vi "ReactorInitialization.vi"(1 "Reactor Selector":T2(ring)) -> (0 "System Constants":T1)   [LabVIEW 2022 SP3]
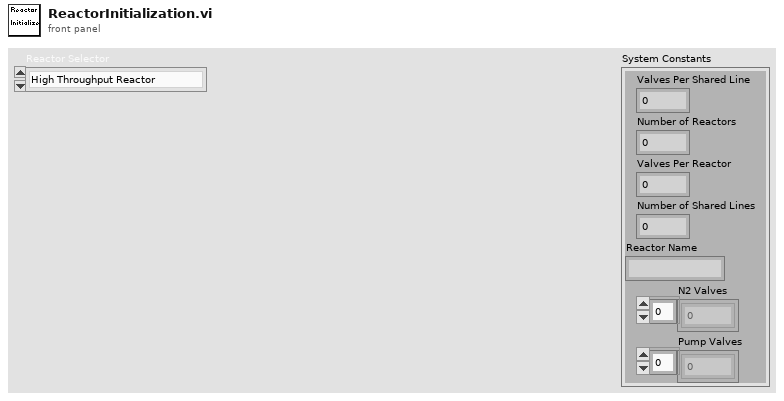
[diagram p1: front panel]
types:
  T1 = cluster{"Valves Per Shared Line":i32, "Number of Reactors":i32, "Valves Per Reactor":i32, "Number of Shared Lines":i32, "Reactor Name":string, "N2 Valves":i32[], "Pump Valves":i32[]}
  T2 = enum16{"High Throughput Reactor", "In Situ Reactor", "MLD Reactor"}
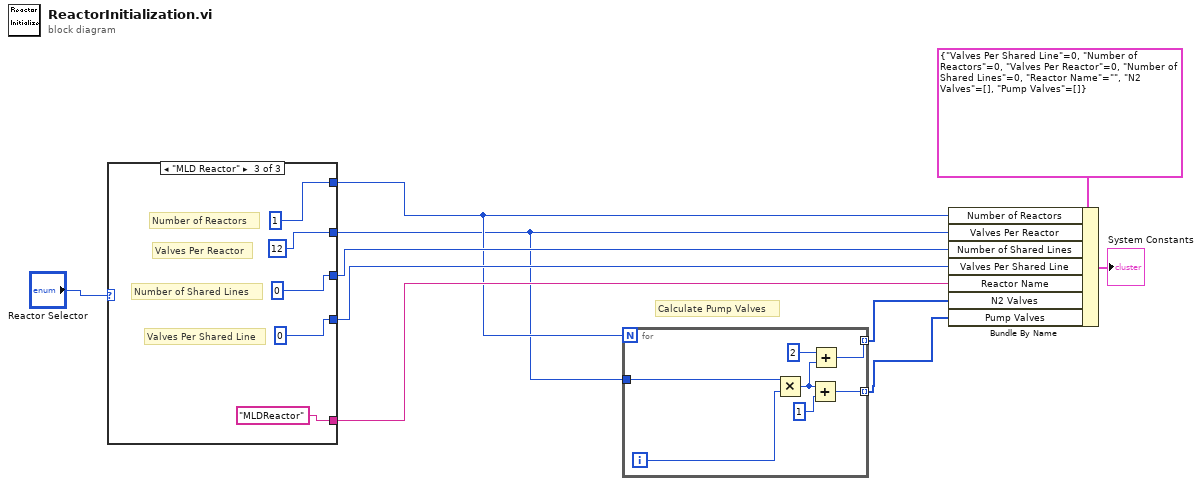
[diagram p0: block diagram]
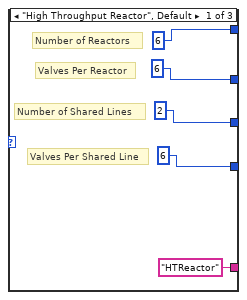
[diagram p2: hidden frame]
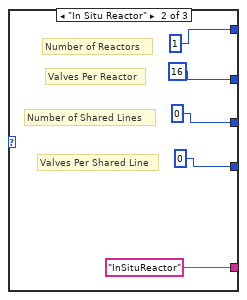
[diagram p3: hidden frame]
diagram:
  # "Calculate Pump Valves"
  n1 = case shown="\"MLD Reactor\"" "Reactor Selector" {
    tunnel: [6 1 1] -> w2
    tunnel: [6 16 12] -> w1
    tunnel: [2 0 0] -> w5
    tunnel: [6 0 0] -> w4
    tunnel: ["HTReactor" ("Reactor Name") "InSituReactor" ("Reactor Name") "MLDReactor" ("Reactor Name")] -> w3
    frame "High Throughput Reactor", Default {
      # "Valves Per Shared Line"
      # "Number of Shared Lines"
      # "Valves Per Reactor"
      # "Number of Reactors"
    }
    frame "In Situ Reactor" {
      # "Valves Per Shared Line"
      # "Number of Shared Lines"
      # "Valves Per Reactor"
      # "Number of Reactors"
    }
    frame "MLD Reactor" {
      # "Valves Per Shared Line"
      # "Number of Shared Lines"
      # "Valves Per Reactor"
      # "Number of Reactors"
    }
  }
  n2 = for {
    N: w2 -> [_]
    tunnel: [w30] -> w7 mode=indexing
    tunnel: [w27] -> w8 mode=indexing
    tunnel: w1 -> [w26]
    i -> [w32]
    n3 = Multiply(x=w26, y=w32) -> (x*y=w29:i32)
    n4 = Add(x=w29, y=1) -> (x+y=w30:i32)
    n5 = Add(x=2, y=w29) -> (x+y=w27:i32)
  }
  n6 = Bundle By Name(cluster=T1 {"Valves Per Shared Line"=0, "Number of Reactors"=0, "Valves Per Reactor"=0, "Number of Shared Lines"=0, "Reactor Name"="", "N2 Valves"=[], "Pump Valves"=[]} ("input cluster"), "Number of Reactors"=w2, "Valves Per Reactor"=w1, "Number of Shared Lines"=w5, "Valves Per Shared Line"=w4, "Reactor Name"=w3, "N2 Valves"=w8, "Pump Valves"=w7) -> (→"System Constants":T1)
